vi "COD读取DATA全局.vi"() -> ()   [LabVIEW 2016, in "斯坦道CODMn.lvlib"]
panel:
  out "配置文件ini":string="data\\Set.ini"
  out "序列号:":string
  out "读取浮台参数显示":bool
  out "读取浮台参数":u16[](array[numeric])
  out "读取公式":u16[](array[numeric])
  out "读取参数":u16[](array[numeric])
  out "数据存储":u16[](array[numeric])
  out "温度":bool[](array[boolean])
  out "M输出点":bool[](array[boolean])
  out "ORP、时间":u16[](array[numeric])
  out "测量状态":u16[](array[numeric])
  out "读取公式显示":bool
  out "读取参数显示":bool
  out "读取写入data":bool
  in  "基本量程存储数据用":enum16{"L", "H"}(ring)
  out "温度存储数据用":dbl
  out "故障标记":bool
  out "数据存储时间戳":timestamp format="%<%Y/%m/%d %H:%M:%S>T"
  out "通讯状态":bool
  out "测量数据区":T1 {"单位" items=["ug/L", "mg/L", "ppm", "mg/m3", "cm", "ppb", "ug/m3", "%", "nmol/mol", "umol/mol", "MPN/L", "MPN/100ml", "ng/m3", "NTU", "无量纲", "ms/cm", "us/cm", "℃", "mV", "万个/L"]}
  out "data":T2
  # "基本量程（20mL可选）："
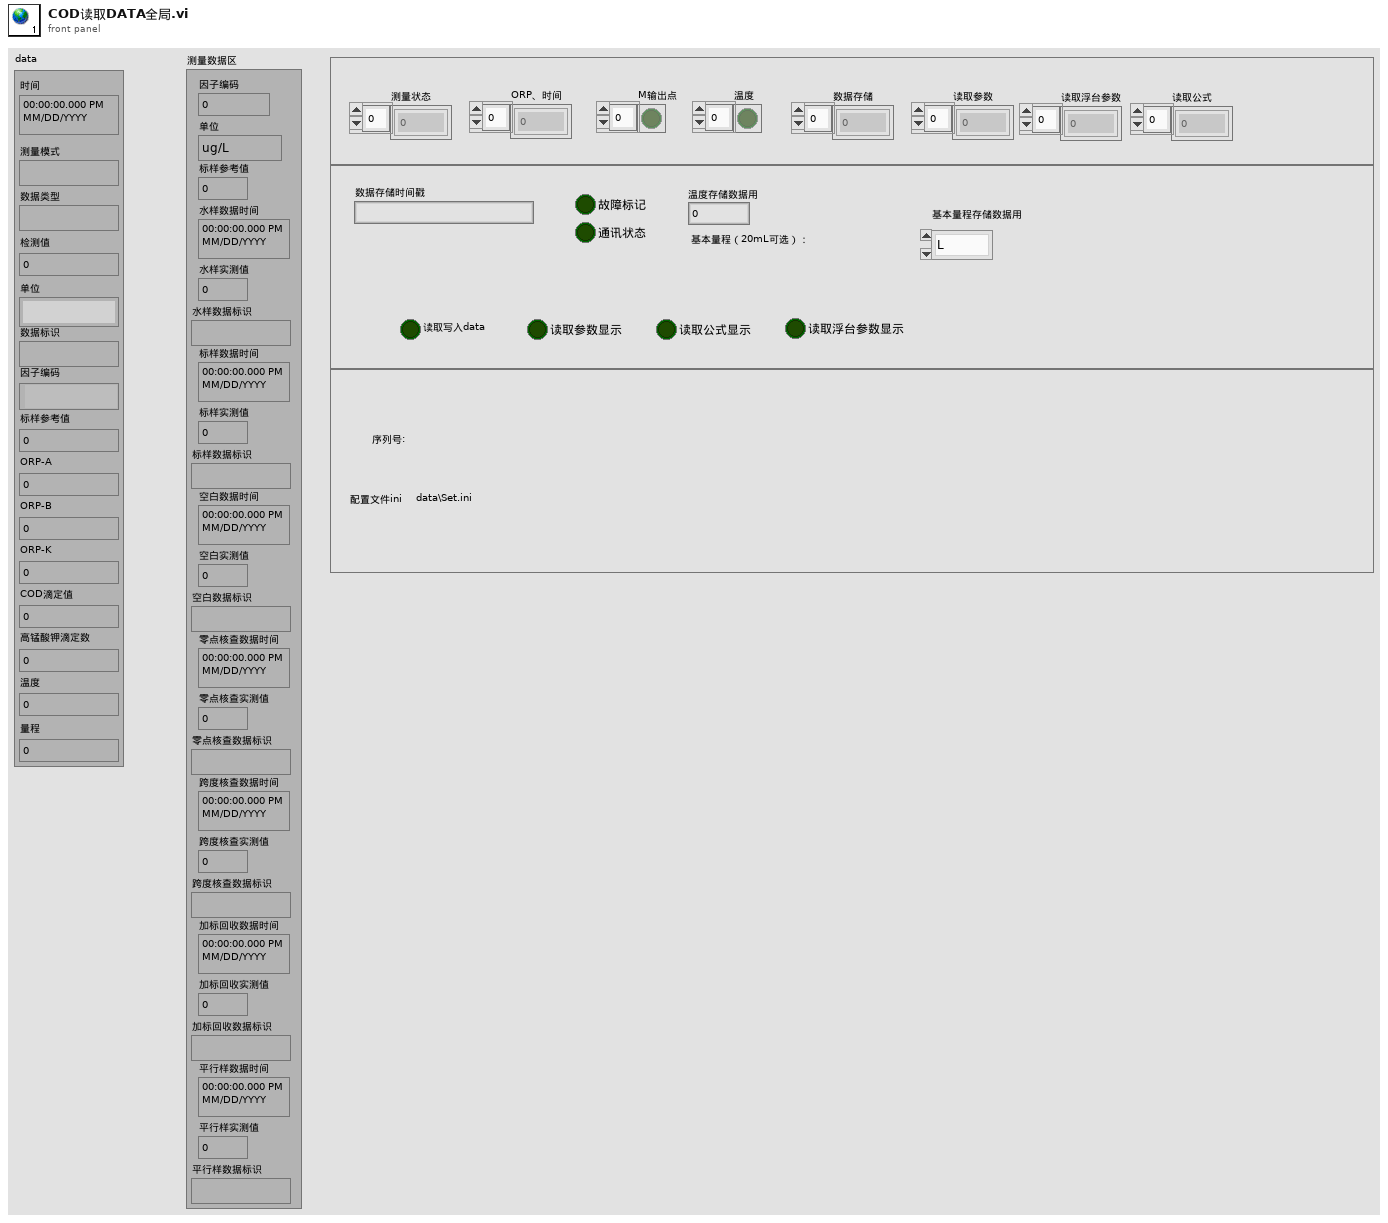
[diagram p1: front panel]
types:
  T1 = cluster{"因子编码":u32, "单位":u16, "标样参考值":sgl, "水样数据时间":timestamp, "水样实测值":sgl, "水样数据标识":string, "标样数据时间":timestamp, "标样实测值":sgl, "标样数据标识":string, "空白数据时间":timestamp, "空白实测值":sgl, "空白数据标识":string, "零点核查数据时间":timestamp, "零点核查实测值":sgl, "零点核查数据标识":string, "跨度核查数据时间":timestamp, "跨度核查实测值":sgl, "跨度核查数据标识":string, "加标回收数据时间":timestamp, "加标回收实测值":sgl, "加标回收数据标识":string, "平行样数据时间":timestamp, "平行样实测值":sgl, "平行样数据标识":string}
  T2 = cluster{"时间":timestamp, "测量模式":string, "数据类型":string, "检测值":sgl, "单位":string, "数据标识":string, "因子编码":string, "标样参考值":sgl, "ORP-A":sgl, "ORP-B":sgl, "ORP-K":sgl, "COD滴定值":sgl, "高锰酸钾滴定数":sgl, "温度":sgl, "量程":sgl}
diagram:
